vi "img test14(manual vs tracked value).vi"() -> ()   [LabVIEW 2014]
uses:
  <vilib>/Utility/sysdir.llb/System Directory Type.ctl
  <vilib>/Utility/file.llb/Write To Spreadsheet File (string).vi
  <vilib>/vision/NI_Vision_Development_Module.lvlib
panel:
  out "Array of Real World Coordinates 2":cluster{"X":sgl, "Y":sgl}[](array[cluster]) {"Y" format="%.2f"; "X" format="%.2f"}
  out "Array of Real World Coordinates":cluster{"X":sgl, "Y":sgl}[](array[cluster]) {"Y" format="%.2f"; "X" format="%.2f"}
  out "Top VIew 3":cluster{"X":sgl, "Y":sgl}[](graph) caption="Top VIew"
  out "ref points":T1
  out "manual bottom 2":T2[](array[typedef]) {"Y" format="%.2f"; "X" format="%.2f"}
  out "manual top 2":T2[](array[typedef]) {"Y" format="%.2f"; "X" format="%.2f"}
  out "Auto bottom 2":cluster{"Numeric":dbl, "Numeric":dbl}[](array[cluster])
  out "Auto top 2":cluster{"Numeric":dbl, "Numeric":dbl}[](array[cluster])
  out "Auto top":cluster{"Numeric":dbl, "Numeric":dbl}[](array[cluster])
  out "manual bottom":T2[](array[typedef]) {"Y" format="%.2f"; "X" format="%.2f"}
  in  "ON":bool
  in  "STOP":bool
  out "appended array":cluster{"Numeric":dbl, "Numeric":dbl}[](array[cluster])
  out "Top VIew 2":cluster{"X":sgl, "Y":sgl}[](graph) caption="Top VIew"
  out "Auto bottom":cluster{"Numeric":dbl, "Numeric":dbl}[](array[cluster])
  out "Point":T2 {"Y" format="%.2f"; "X" format="%.2f"}
  out "manual top":T2[](array[typedef]) {"Y" format="%.2f"; "X" format="%.2f"}
  out "Number of Frames":u32
  out "Top player court segment display 2":bool[][](array[boolean])
  out "count top":i32[](graph)
  out "count bottom":i32[](graph)
  out "trans top":i32[](graph)
  out "trans bottom":i32[](graph)
  out "trans array bottom":i32[](array[numeric])
  out "trans array top":i32[](array[numeric])
  out "count array bottom":i32[](array[numeric])
  out "Count array top":i32[](array[numeric])
  in  "ON":bool
  out "Top player court segment display":bool[][](array[boolean])
  out "bottom player":cluster{"Numeric":dbl, "Numeric":dbl}[](array[cluster])
  out "top player":cluster{"Numeric":dbl, "Numeric":dbl}[](array[cluster])
  in  "playing":bool
  out "Top VIew":cluster{"Numeric":dbl, "Numeric":dbl}[](graph)
  out "Image 4":T3(plugin-control)
  in  "frame jump":i32=3
  in  "speed":u32(slide)
  in  "start":i32(slide) step=219843704 scale=0.0..62085.0
  out "Image 3":T3(plugin-control)
  in  "AVI Path":path=path "E:/PhD work/PhD research work/Videos/Chen Jin vs Hu Yun (Edited).avi"
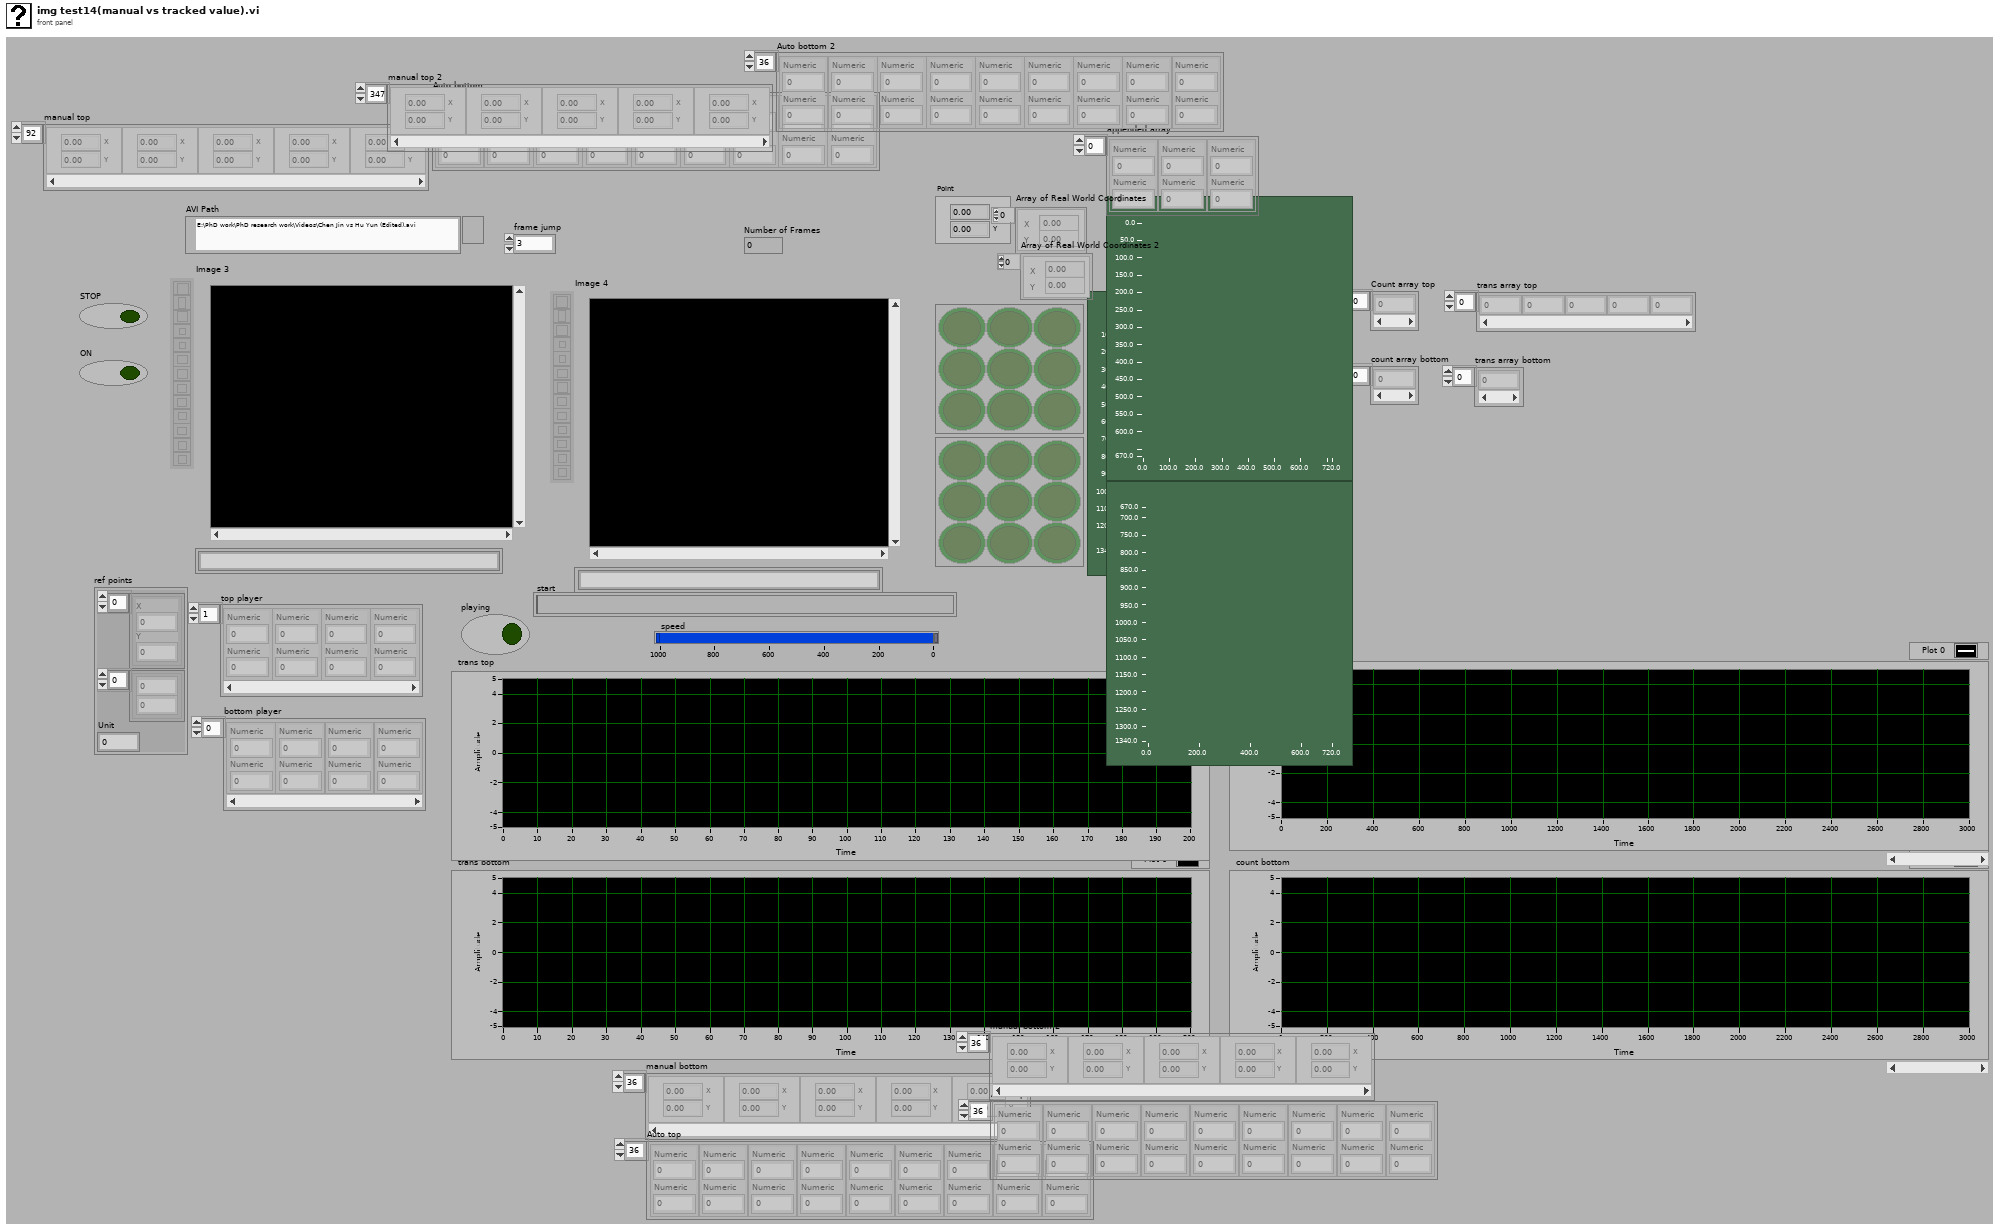
[diagram p1: front panel]
types:
  T1 = cluster{cluster{"X":sgl, "Y":sgl}[], cluster{i32, i32}[], "Unit":u32}
  T2 = typedef "IMAQ Point" = cluster{"X":sgl, "Y":sgl}
  T3 = typedef "IMAQ Image.ctl" = refnum<image>
  T4 = typedef "System Directory Type.ctl" = i32
  T5 = cluster{"Origin Pixel":cluster{"X":sgl, "Y":sgl}, "Angle Relative to Horizontal (deg)":sgl, "Axis Reference":u32}
  T6 = typedef "Image Type" = u32
  T7 = typedef "AviRefnum.ctl" = refnum<k1>
  T8 = cluster{"width":u32, "height":u32, "framesPerSecond":u32, "compressionFilter":string, "hasData":bool}
  T9 = typedef "Particle Parameters" = i32
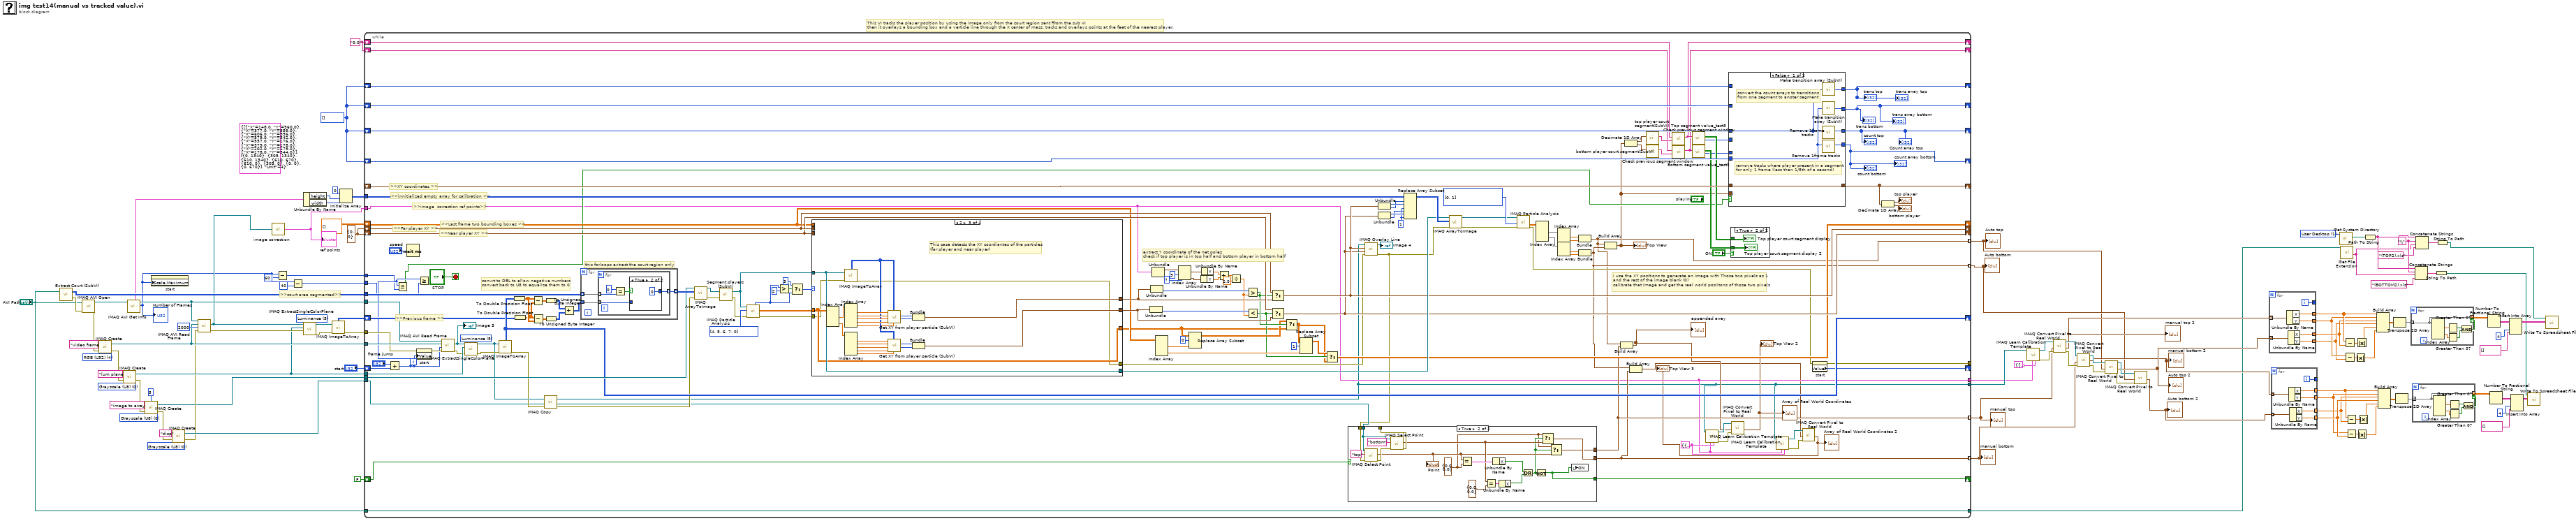
[diagram p0: block diagram]
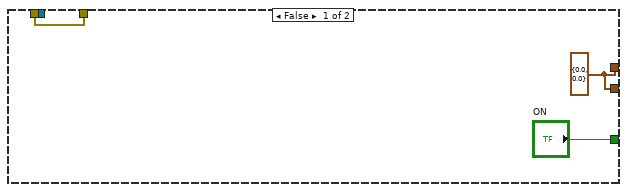
[diagram p2: hidden frame]
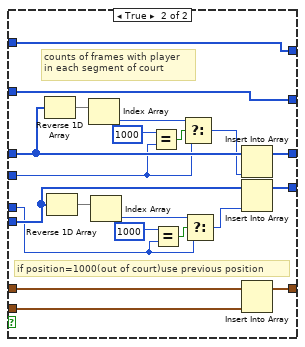
[diagram p3: hidden frame]
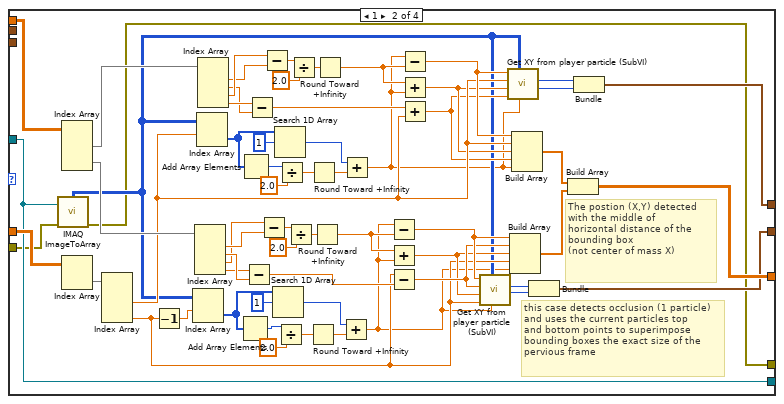
[diagram p6: hidden frame]
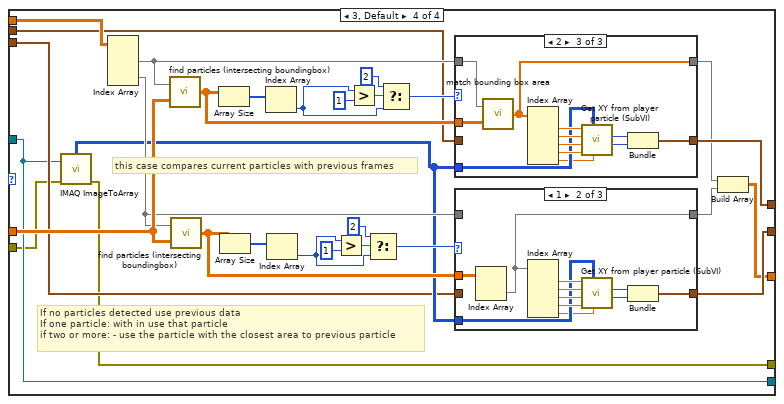
[diagram p7: hidden frame]
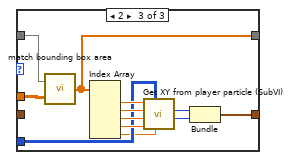
[diagram p9: hidden frame]
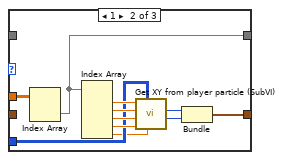
[diagram p11: hidden frame]
diagram:
  w7 = "\\" ("string")
  w17 = T4 1 items=["User Home"=0, "User Desktop"=1, "User Documents"=2, "User Application Data"=3, "User Preferences"=4, "User Temporary"=5, "Public Documents"=6, "Public Application Data"=7, "Public Preferences"=8, "Public Cache"=13, "System Core Libraries"=9, "System Installed Libraries"=10, "Application Files"=11, "Boot Volume Root"=12] ("system directory type")
  (unwired) T1 {[{"X"=148.0, "Y"=560.0}, {"X"=377.0, "Y"=559.0}, {"X"=606.0, "Y"=556.0}, {"X"=579.0, "Y"=342.0}, {"X"=557.0, "Y"=176.0}, {"X"=379.0, "Y"=178.0}, {"X"=202.0, "Y"=179.0}, {"X"=178.0, "Y"=344.0}], [{0, 1340}, {305, 1340}, {610, 1340}, {610, 670}, {610, 0}, {305, 0}, {0, 0}, {0, 670}], "Unit"=4} ("ref points")
  w71 = "0,0" ("Player segment position")
  w72 = i32[] [] ("input array")
  w82 = cluster{"X coordinate":i32, "Y coordinate":i32} {"X coordinate"=0, "Y coordinate"=0}
  w95 = T6 0 items=["Grayscale (U8)", "Grayscale (I16)", "Grayscale (SGL)", "Complex (CSG)", "RGB (U32)", "HSL (U32)", "RGB (U64)", "Grayscale (U16)"] ("Image Type")
  w102 = 5 items=["Red", "Green", "Blue", "Hue", "Saturation", "Luminance", "Value", "Intensity"] ("Color Plane")
  w103 = T6 0 items=["Grayscale (U8)", "Grayscale (I16)", "Grayscale (SGL)", "Complex (CSG)", "RGB (U32)", "HSL (U32)", "RGB (U64)", "Grayscale (U16)"] ("Image Type")
  w107 = T6 0 items=["Grayscale (U8)", "Grayscale (I16)", "Grayscale (SGL)", "Complex (CSG)", "RGB (U32)", "HSL (U32)", "RGB (U64)", "Grayscale (U16)"] ("Image Type")
  w105 = T6 4 items=["Grayscale (U8)", "Grayscale (I16)", "Grayscale (SGL)", "Complex (CSG)", "RGB (U32)", "HSL (U32)", "RGB (U64)", "Grayscale (U16)"] ("Image Type")
  # ">>court area segmented>>"
  # "This VI tracks the player position by using the image only from the court region sent ffrom the sub VI\nthen it overlays a bounding box and a verticle line through the X center of mass. tracks and overlays points at the feet of the nearest player."
  n1 = call "Extract Court (SubVI).vi"("AVI Path"="AVI Path") -> ("error out"=w109:errorcluster, "Court pixels out"=w85:u8[][])  [unwired: 1 in]
  n2 = call "IMAQ AVI Open"("error in (no error)"=w109, "AVI Path"="AVI Path") -> ("error out"=w91:errorcluster, "Avi Refnum"=w80:T7)  [unwired: 8 in]
  n3 = call "IMAQ Create"("Image Name"="video frame", "Image Type"=w105, "error in (no error)"=w91) -> ("New Image"=w99:T3, "error out"=w90:errorcluster)  [unwired: 2 in]
  n4 = call "IMAQ Create"("Image Name"="lum plane", "Image Type"=w107, "error in (no error)"=w90) -> ("New Image"=w98:T3, "error out"=w89:errorcluster)  [unwired: 2 in]
  n5 = call "IMAQ AVI Get Info"("Avi Refnum"=w80) -> ("Number of Frames"=w69:u32, "Avi Refnum (duplicate)"=w79:T7, "Frame Data"=w76:T8)  [unwired: 6 in, 2 out]
  "Number of Frames" <- w69
  n6 = call "IMAQ Create"("Border Size"=5, "Image Name"="image to array", "Image Type"=w103, "error in (no error)"=w89) -> ("New Image"=w84:T3, "error out"=w88:errorcluster)  [unwired: 1 in]
  n7 = property on="start" class="Slide (strict)"("Scale.Maximum"=w69) -> ()  [unwired: 2 in, 2 out]
  n8 = call "IMAQ Create"("Image Name"="disp", "Image Type"=w95, "error in (no error)"=w88) -> ("New Image"=w93:T3, "error out"=w87:errorcluster)  [unwired: 2 in]
  n9 = call "IMAQ AVI Read Frame"("error in (no error)"=w87, "Frame Number"=u32 2000, "Image"=w99, "Avi Refnum"=w79) -> ("error out"=w101:errorcluster, "Image Out"=w70:T3)  [unwired: 4 in, 2 out]
  n10 = call "image correction.vi"("Image"=w70) -> ("ref points"=w1:T1)
  "ref points" <- w1
  n11 = Subtract(x=w69, y=u32 60) -> (x-y=w66:u32)
  n12 = Subtract(x=w69, y=u32 40) -> (x-y=w65:u32)
  n13 = Unbundle By Name(w76) -> ("height"=w75:u32, "width"=w74:u32)
  n14 = call "IMAQ ExtractSingleColorPlane"("Color Plane"=w102, "error in (no error)"=w101, "Image Dst"=w98, "Image Src"=w70) -> ("error out"=w92:errorcluster, "Image Dst Out"=w96:T3)  [unwired: 6 in]
  n15 = call "IMAQ ImageToArray"("error in (no error)"=w92, "Image"=w96) -> ("error out"=w78:errorcluster, "Image Pixels (U8)"=w97:u8[][])  [unwired: 2 in, 3 out]
  n16 = Initialize Array(u8 0 ("element"), w75, w74) -> (w73:u8[][])
  n17 = while {
    tunnel: w79 -> [w219]
    tunnel: w99 -> [w236]
    tunnel: w85 -> [w251]
    tunnel: w98 -> [w237]
    tunnel: w84 -> [w249]
    shift-right: [w248] -> _
    shift-left: w97 -> [w247]
    tunnel: w93 -> [w127]
    shift-right: [w168] -> _
    shift-left: dbl[][] [] ("Particle Measurements (Pixels)") -> [w178]
    shift-right: [w182] -> _
    shift-left: w82 -> [w184]
    shift-right: [w180] -> _
    shift-left: w82 -> [w183]
    shift-right: [w216] -> _
    shift-left: "start" -> [w221]
    tunnel: w78 -> [w218]
    tunnel: w73 -> [w215]
    tunnel: w1 -> [w115]
    shift-right: [w154] -> _
    shift-left: _ -> [w199]
    shift-right: [w152] -> _
    shift-left: w72 -> [w157]
    shift-right: [w151] -> _
    shift-left: w72 -> [w158]
    tunnel: [w160] -> _
    shift-right: [w144] -> _
    shift-left: w72 -> [w155]
    shift-right: [w153] -> _
    shift-left: w72 -> [w156]
    shift-right: [w138] -> _
    shift-left: w71 -> [w145]
    shift-right: [w139] -> _
    shift-left: w71 -> [w146]
    tunnel: w66 -> [w137]
    tunnel: w65 -> [w136]
    tunnel: [w133] -> w5 mode=indexing
    tunnel: [w125] -> w3 mode=indexing
    shift-right: [w129] -> _
    shift-left: FALSE ("ON") -> [w128]
    tunnel: [w123] -> w4 mode=indexing
    tunnel: [w124] -> w2 mode=indexing
    tunnel: [w114] -> w63
    tunnel: [w115] -> w62
    tunnel: "AVI Path" -> [w126]
    tunnel: [w126] -> w15
    stop <- "STOP" stop-if-true
    w116 = T5 {"Origin Pixel"={"X"=-1.0, "Y"=-1.0}, "Angle Relative to Horizontal (deg)"=0.0, "Axis Reference"=1} ("Calibration Axis Info")
    w207 = T9[] [0, 1] items=["Center of Mass X", "Center of Mass Y", "First Pixel X", "First Pixel Y", "Bounding Rect Left", "Bounding Rect Top", "Bounding Rect Right", "Bounding Rect Bottom", "Max Feret Diameter Start X", "Max Feret Diameter Start Y", "Max Feret Diameter End X", "Max Feret Diameter End Y", "Max Horiz. Segment Length Left", "Max Horiz. Segment Length Right", "Max Horiz. Segment Length Row", "-", "Bounding Rect Width", "Bounding Rect Height", "Bounding Rect Diagonal", "Perimeter", "Convex Hull Perimeter", "Holes' Perimeter", "Max Feret Diameter", "Equivalent Ellipse Major Axis", "Equivalent Ellipse Minor Axis", "Equivalent Ellipse Minor Axis (Feret)", "Equivalent Rect Long Side", "Equivalent Rect Short Side", "Equivalent Rect Diagonal", "Equivalent Rect Short Side (Feret)", "Average Horiz. Segment Length", "Average Vert. Segment Length", "Hydraulic Radius", "Waddel Disk Diameter", "-", "Area", "Holes' Area", "Particle & Holes' Area", "Convex Hull Area", "Image Area", "-", "Number of Holes", "Number of Horiz. Segments", "Number of Vert. Segments", "-", "Orientation", "Max Feret Diameter Orientation", "-", "% Area/Image Area", "% Area/(Particle & Holes' Area)", "Ratio of Equivalent Ellipse Axes", "Ratio of Equivalent Rect Sides", "-", "Elongation Factor", "Compactness Factor", "Heywood Circularity Factor", "Type Factor", "-", "Sum X", "Sum Y", "Sum XX", "Sum XY", "Sum YY", "Sum XXX", "Sum XXY", "Sum XYY", "Sum YYY", "-", "Moment of Inertia XX", "Moment of Inertia XY", "Moment of Inertia YY", "Moment of Inertia XXX", "Moment of Inertia XXY", "Moment of Inertia XYY", "Moment of Inertia YYY", "Norm. Moment of Inertia XX", "Norm. Moment of Inertia XY", "Norm. Moment of Inertia YY", "Norm. Moment of Inertia XXX", "Norm. Moment of Inertia XXY", "Norm. Moment of Inertia XYY", "Norm. Moment of Inertia YYY", "Hu Moment 1", "Hu Moment 2", "Hu Moment 3", "Hu Moment 4", "Hu Moment 5", "Hu Moment 6", "Hu Moment 7"] ("Real-World Measurements")
    w210 = u8 1 ("new element/subarray")
    w238 = T9[] [4, 5, 6, 7, 0] items=["Center of Mass X", "Center of Mass Y", "First Pixel X", "First Pixel Y", "Bounding Rect Left", "Bounding Rect Top", "Bounding Rect Right", "Bounding Rect Bottom", "Max Feret Diameter Start X", "Max Feret Diameter Start Y", "Max Feret Diameter End X", "Max Feret Diameter End Y", "Max Horiz. Segment Length Left", "Max Horiz. Segment Length Right", "Max Horiz. Segment Length Row", "-", "Bounding Rect Width", "Bounding Rect Height", "Bounding Rect Diagonal", "Perimeter", "Convex Hull Perimeter", "Holes' Perimeter", "Max Feret Diameter", "Equivalent Ellipse Major Axis", "Equivalent Ellipse Minor Axis", "Equivalent Ellipse Minor Axis (Feret)", "Equivalent Rect Long Side", "Equivalent Rect Short Side", "Equivalent Rect Diagonal", "Equivalent Rect Short Side (Feret)", "Average Horiz. Segment Length", "Average Vert. Segment Length", "Hydraulic Radius", "Waddel Disk Diameter", "-", "Area", "Holes' Area", "Particle & Holes' Area", "Convex Hull Area", "Image Area", "-", "Number of Holes", "Number of Horiz. Segments", "Number of Vert. Segments", "-", "Orientation", "Max Feret Diameter Orientation", "-", "% Area/Image Area", "% Area/(Particle & Holes' Area)", "Ratio of Equivalent Ellipse Axes", "Ratio of Equivalent Rect Sides", "-", "Elongation Factor", "Compactness Factor", "Heywood Circularity Factor", "Type Factor", "-", "Sum X", "Sum Y", "Sum XX", "Sum XY", "Sum YY", "Sum XXX", "Sum XXY", "Sum XYY", "Sum YYY", "-", "Moment of Inertia XX", "Moment of Inertia XY", "Moment of Inertia YY", "Moment of Inertia XXX", "Moment of Inertia XXY", "Moment of Inertia XYY", "Moment of Inertia YYY", "Norm. Moment of Inertia XX", "Norm. Moment of Inertia XY", "Norm. Moment of Inertia YY", "Norm. Moment of Inertia XXX", "Norm. Moment of Inertia XXY", "Norm. Moment of Inertia XYY", "Norm. Moment of Inertia YYY", "Hu Moment 1", "Hu Moment 2", "Hu Moment 3", "Hu Moment 4", "Hu Moment 5", "Hu Moment 6", "Hu Moment 7"] ("Pixel Measurements")
    w252 = 5 items=["Red", "Green", "Blue", "Hue", "Saturation", "Luminance", "Value", "Intensity"] ("Color Plane")
    # ">>XY coordinates >>"
    # ">>innitialized empty array for calibration >>"
    # ">>image  correction ref points>>"
    # "extract Y coordinate of the net poles\ncheck if top player is in top half and bottom player in bottom half"
    # "i use the XY positions to generate an Image with Those two pixels as 1 \nand the rest of the image blank (0)\ncalibrate that image and get the real world posiitons of those two pixels"
    # ">>Last frame two bounding boxes >>"
    # ">>Far player XY >>"
    # ">>Near player XY >>"
    # ">>Previous frame >>"
    # "convrt to DBL to allow negative numbers\nconvert back to U8 to equalize them to 0"
    # "this forloops extract the court region only"
    n18 = Add(x="frame jump", y=w221) -> (x+y=w143:i32)
    n19 = Less Or Equal?(x=w143, y=w137) -> (x <= y?=w142:bool)
    n20 = Wait (ms)(milliseconds to wait="speed") -> ()  [unwired: 1 out]
    n21 = property on="start" class="Slide (strict)"(error in=w218, "Value"=w143) -> (error out=w217:errorcluster)  [unwired: 1 in, 1 out]
    n22 = Greater Or Equal?(x=w143, y=w136) -> ()  [unwired: 1 out]
    n23 = call "IMAQ AVI Read Frame"("error in (no error)"=w217, "Frame Number"=w143, "Image"=w236, "Avi Refnum"=w219) -> ("error out"=w111:errorcluster, "Image Out"=w135:T3)  [unwired: 4 in, 2 out]
    "Image 3" <- w135
    n24 = call "IMAQ ExtractSingleColorPlane"("Color Plane"=w252, "error in (no error)"=w111, "Image Dst"=w237, "Image Src"=w135) -> ("error out"=w239:errorcluster, "Image Dst Out"=w222:T3)  [unwired: 6 in]
    n25 = call "IMAQ ImageToArray"("error in (no error)"=w239, "Image"=w222) -> ("error out"=w164:errorcluster, "Image Pixels (U8)"=w248:u8[][])  [unwired: 2 in, 3 out]
    n26 = To Double Precision Float(number=w248) -> (double precision float=w243:dbl[][])
    n27 = To Double Precision Float(number=w247) -> (double precision float=w242:dbl[][])
    n28 = Subtract(x=w243, y=w242) -> (x-y=w241:dbl[][])
    n29 = Subtract(x=w242, y=w243) -> (x-y=w240:dbl[][])
    n30 = call "IMAQ Copy"("error in (no error)"=w164, "Image Dst"=w127, "Image Src"=w222) -> ("error out"=w163:errorcluster, "Image Dst Out"=w114:T3)  [unwired: 3 in]
    n31 = To Unsigned Byte Integer(number=w241) -> (unsigned 8bit integer=w246:u8[][])
    n32 = To Unsigned Byte Integer(number=w240) -> (unsigned 8bit integer=w245:u8[][])
    n33 = Add(x=w246, y=w245) -> (x+y=w244:u8[][])
    n34 = for {
      tunnel: w251 -> [w474] mode=indexing
      tunnel: [w473] -> w250 mode=indexing
      tunnel: w244 -> [w472] mode=indexing
      n35 = for {
        tunnel: w474 -> [w479] mode=indexing
        tunnel: [w476] -> w473 mode=indexing
        tunnel: w472 -> [w475] mode=indexing
        n36 = Equal?(x=u8 0, y=w479) -> (x = y?=w477:bool)
        n37 = case shown="True" w477 {
          tunnel: [w480 u8 0 ("x")] -> w476
          tunnel: w475 -> [w480 _]
          frame False {
          }
          frame True {
          }
        }
      }
    }
    n38 = call "IMAQ ArrayToImage"("error in (no error)"=w163, "Image Pixels (U8)"=w250, "Image"=w249) -> ("error out"=w234:errorcluster, "Image Out"=w235:T3)  [unwired: 7 in]
    n39 = call "Segment players (SubVI).vi"("error In"=w234, "Image In"=w235) -> ("error out"=w228:errorcluster, "Image Out"=w226:T3)
    n40 = call "IMAQ Particle Analysis"("error in (no error)"=w228, "Pixel Measurements"=w238, "Image"=w226) -> ("error out"=w227:errorcluster, "Particle Measurements (Pixels)"=w225:dbl[][], "Number of Particles"=w230:i32)  [unwired: 3 in, 3 out]
    n41 = Greater?(x=w230, y=2) -> (0:w233:bool)
    n42 = Select(t=3 ("y"), s=w233, f=w230) -> (s? t:f=w229:i32)
    n43 = case shown="2" w229 {
      tunnel: [w307 w334 w388 w398] -> w208
      tunnel: w225 -> [_ w369 w374 w418]
      tunnel: w227 -> [w304 w310 w371 w394]
      tunnel: w226 -> [w307 w334 w388 w398]
      tunnel: [w305 w318 w376 w400] -> w179
      tunnel: [w306 w325 w375 w399] -> w181
      tunnel: [w308 w335 w374 w395] -> w167
      tunnel: w178 -> [w308 w359 _ w421]
      tunnel: w184 -> [w306 _ _ w406]
      tunnel: w183 -> [w305 _ _ w401]
      tunnel: [w304 w309 w370 w393] -> w162
      frame 0 {
        # "This case identifies frames where no particles are detected and keeps the same values from the\nprevious frame"
      }
      frame 1 {
        # "The postion (X,Y) detected with the middle of \nhorizontal distance of the bounding box\n(not center of mass X)"
        # "this case detects occlusion (1 particle)\nand uses the current particles top \nand bottom points to superimpose \nbounding boxes the exact size of the \npervious frame"
        n44 = call "IMAQ ImageToArray"("error in (no error)"=w310, "Image"=w334) -> ("error out"=w309:errorcluster, "Image Pixels (U8)"=w317:u8[][])  [unwired: 2 in, 3 out]
        n45 = Index Array(array=w359) -> (element #1=w367:dbl[], element #2=w339:dbl[])  [unwired: 4 in]
        n46 = Index Array(array=w369) -> (element=w368:dbl[])  [unwired: 2 in]
        n47 = Index Array(array=w368) -> (element #2=w330:dbl, element #4=w321:dbl)  [unwired: 4 in, 2 out]
        n48 = Decrement(x=w321) -> (x-1=w332:dbl)
        n49 = Index Array(array=w317, index (row)=w332) -> (element=w354:u8[])  [unwired: 1 in]
        n50 = Index Array(array=w339) -> (element #1=w343:dbl, element #2=w346:dbl, element #3=w342:dbl, element #4=w345:dbl)  [unwired: 4 in]
        n51 = Index Array(array=w317, index (row)=w330) -> (element=w347:u8[])  [unwired: 1 in]
        n52 = Index Array(array=w367) -> (element #1=w363:dbl, element #2=w360:dbl, element #3=w364:dbl, element #4=w361:dbl)  [unwired: 4 in]
        n53 = Add Array Elements(numeric array=w354) -> (sum=w355:u8)
        n54 = Add Array Elements(numeric array=w347) -> (sum=w351:u8)
        n55 = Subtract(x=w345, y=w346) -> (x-y=w333:dbl)
        n56 = Subtract(x=w361, y=w360) -> (x-y=w338:dbl)
        n57 = Subtract(x=w342, y=w343) -> (x-y=w341:dbl)
        n58 = Subtract(x=w364, y=w363) -> (x-y=w365:dbl)
        n59 = Search 1D Array(1D array=w354, element=u8 1) -> (index of element=w353:i32)  [unwired: 1 in]
        n60 = Search 1D Array(1D array=w347, element=u8 1) -> (index of element=w352:i32)  [unwired: 1 in]
        n61 = Divide(x=w355, y=2.0) -> (x/y=w356:dbl)
        n62 = Divide(x=w351, y=2.0) -> (x/y=w350:dbl)
        n63 = Divide(x=w341, y=2.0) -> (x/y=w344:dbl)
        n64 = Divide(x=w365, y=2.0) -> (x/y=w362:dbl)
        n65 = Round Toward +Infinity(x=w356) -> (ceil(x): smallest int >= x=w315:dbl)
        n66 = Round Toward +Infinity(x=w350) -> (ceil(x): smallest int >= x=w314:dbl)
        n67 = Round Toward +Infinity(x=w344) -> (ceil(x): smallest int >= x=w316:dbl)
        n68 = Round Toward +Infinity(x=w362) -> (ceil(x): smallest int >= x=w313:dbl)
        n69 = Add(x=w353, y=w315) -> (x+y=w311:dbl)
        n70 = Add(x=w352, y=w314) -> (x+y=w312:dbl)
        n71 = Subtract(x=w311, y=w316) -> (x-y=w324:dbl)
        n72 = Add(x=w316, y=w311) -> (x+y=w322:dbl)
        n73 = Subtract(x=w321, y=w333) -> (x-y=w323:dbl)
        n74 = Subtract(x=w312, y=w313) -> (x-y=w331:dbl)
        n75 = Add(x=w313, y=w312) -> (x+y=w329:dbl)
        n76 = Add(x=w338, y=w330) -> (x+y=w328:dbl)
        n77 = call "Get XY from player particle (SubVI).vi"("Center of mass X"=w311, "Image in Pixels (U8)"=w317, "Particle bounding rect bottom"=w321, "Particle bounding rect right"=w322, "Particle bounding rect top"=w323, "Particle bounding rect left"=w324) -> ("Y coordinate"=w319:i32, "X coordinate"=w320:i32)  [unwired: 2 in]
        n78 = call "Get XY from player particle (SubVI).vi"("Center of mass X"=w312, "Image in Pixels (U8)"=w317, "Particle bounding rect bottom"=w328, "Particle bounding rect right"=w329, "Particle bounding rect top"=w330, "Particle bounding rect left"=w331) -> ("Y coordinate"=w326:i32, "X coordinate"=w327:i32)  [unwired: 2 in]
        n79 = Build Array(w324, w323, w322, w321, w311) -> (w336:dbl[])
        n80 = Build Array(w331, w330, w329, w328, w312) -> (w337:dbl[])
        n81 = Bundle("X coordinate"=w320, "Y coordinate"=w319) -> (w318:cluster{"X coordinate":i32, "Y coordinate":i32})  [unwired: 1 in]
        n82 = Build Array(w337, w336) -> (w335:dbl[][])
        n83 = Bundle("X coordinate"=w327, "Y coordinate"=w326) -> (w325:cluster{"X coordinate":i32, "Y coordinate":i32})  [unwired: 1 in]
      }
      frame 2 {
        # "This case detects the XY coordiantes of the particles\n(far player and near player)"
        n84 = Index Array(array=w374) -> (element #1=w382:dbl[], element #2=w381:dbl[])  [unwired: 4 in]
        n85 = call "IMAQ ImageToArray"("error in (no error)"=w371, "Image"=w388) -> ("error out"=w370:errorcluster, "Image Pixels (U8)"=w383:u8[][])  [unwired: 2 in, 3 out]
        n86 = Index Array(array=w382) -> (element #1=w392:dbl, element #2=w391:dbl, element #3=w390:dbl, element #4=w389:dbl, element #5=w373:dbl)  [unwired: 5 in]
        n87 = Index Array(array=w381) -> (element #1=w384:dbl, element #2=w385:dbl, element #3=w386:dbl, element #4=w387:dbl, element #5=w372:dbl)  [unwired: 5 in]
        n88 = call "Get XY from player particle (SubVI).vi"("Center of mass X"=w373, "Image in Pixels (U8)"=w383, "Particle bounding rect bottom"=w389, "Particle bounding rect right"=w390, "Particle bounding rect top"=w391, "Particle bounding rect left"=w392) -> ("Y coordinate"=w379:i32, "X coordinate"=w380:i32)  [unwired: 2 in]
        n89 = call "Get XY from player particle (SubVI).vi"("Center of mass X"=w372, "Image in Pixels (U8)"=w383, "Particle bounding rect bottom"=w387, "Particle bounding rect right"=w386, "Particle bounding rect top"=w385, "Particle bounding rect left"=w384) -> ("Y coordinate"=w377:i32, "X coordinate"=w378:i32)  [unwired: 2 in]
        n90 = Bundle("X coordinate"=w380, "Y coordinate"=w379) -> (w375:cluster{"X coordinate":i32, "Y coordinate":i32})  [unwired: 1 in]
        n91 = Bundle("X coordinate"=w378, "Y coordinate"=w377) -> (w376:cluster{"X coordinate":i32, "Y coordinate":i32})  [unwired: 1 in]
      }
      frame 3, Default {
        # "If no particles detected use previous data\nIf one particle: with in use that particle\nif two or more: - use the particle with the closest area to previous particle"
        # "this case compares current particles with previous frames"
        n92 = call "IMAQ ImageToArray"("error in (no error)"=w394, "Image"=w398) -> ("error out"=w393:errorcluster, "Image Pixels (U8)"=w402:u8[][])  [unwired: 2 in, 3 out]
        n93 = Index Array(array=w421) -> (element #1=w417:dbl[], element #2=w405:dbl[])  [unwired: 4 in]
        n94 = call "find particles (intersecting boundingbox).vi"("Particle Measurements in (bounding boxes)"=w418, "bounding box in"=w417) -> ("Particles within bounding box"=w416:dbl[][])
        n95 = call "find particles (intersecting boundingbox).vi"("Particle Measurements in (bounding boxes)"=w418, "bounding box in"=w405) -> ("Particles within bounding box"=w403:dbl[][])
        n96 = Array Size(array=w416) -> (size(s)=w420:i32[])
        n97 = Array Size(array=w403) -> (size(s)=w419:i32[])
        n98 = Index Array(array=w420) -> (element=w408:i32)  [unwired: 1 in]
        n99 = Index Array(array=w419) -> (element=w409:i32)  [unwired: 1 in]
        n100 = Greater?(x=w409, y=1) -> (0:w412:bool)
        n101 = Greater?(x=w408, y=1) -> (0:w413:bool)
        n102 = Select(t=2 ("y"), s=w412, f=w409) -> (s? t:f=w404:i32)
        n103 = Select(t=2 ("y"), s=w413, f=w408) -> (s? t:f=w407:i32)
        n104 = case shown="2" w407 {
          tunnel: w417 -> [w448 _ w463]
          tunnel: w416 -> [_ w459 w462]
          tunnel: [w448 w450 w461] -> w397
          tunnel: w402 -> [_ w452 w465]
          tunnel: [w447 w451 w464] -> w399
          tunnel: w406 -> [w447 _ _]
          frame 0, Default {
          }
          frame 1 {
            n105 = Index Array(array=w459) -> (element=w450:dbl[])  [unwired: 2 in]
            n106 = Index Array(array=w450) -> (element #1=w456:dbl, element #2=w455:dbl, element #3=w454:dbl, element #4=w453:dbl, element #5=w449:dbl)  [unwired: 5 in]
            n107 = call "Get XY from player particle (SubVI).vi"("Center of mass X"=w449, "Image in Pixels (U8)"=w452, "Particle bounding rect bottom"=w453, "Particle bounding rect right"=w454, "Particle bounding rect top"=w455, "Particle bounding rect left"=w456) -> ("Y coordinate"=w457:i32, "X coordinate"=w458:i32)  [unwired: 2 in]
            n108 = Bundle("X coordinate"=w458, "Y coordinate"=w457) -> (w451:cluster{"X coordinate":i32, "Y coordinate":i32})  [unwired: 1 in]
          }
          frame 2 {
            n109 = call "match bounding box area.vi"("particle measurements (bounding box)"=w462, "bounding box in"=w463) -> ("matching bounding box"=w461:dbl[])
            n110 = Index Array(array=w461) -> (element #1=w469:dbl, element #2=w468:dbl, element #3=w467:dbl, element #4=w466:dbl, element #5=w460:dbl)  [unwired: 5 in]
            n111 = call "Get XY from player particle (SubVI).vi"("Center of mass X"=w460, "Image in Pixels (U8)"=w465, "Particle bounding rect bottom"=w466, "Particle bounding rect right"=w467, "Particle bounding rect top"=w468, "Particle bounding rect left"=w469) -> ("Y coordinate"=w470:i32, "X coordinate"=w471:i32)  [unwired: 2 in]
            n112 = Bundle("X coordinate"=w471, "Y coordinate"=w470) -> (w464:cluster{"X coordinate":i32, "Y coordinate":i32})  [unwired: 1 in]
          }
        }
        n113 = case shown="1" w404 {
          tunnel: w405 -> [w423 _ w438]
          tunnel: w403 -> [_ w434 w437]
          tunnel: [w423 w425 w436] -> w396
          tunnel: w402 -> [_ w427 w440]
          tunnel: [w422 w426 w439] -> w400
          tunnel: w401 -> [w422 _ _]
          frame 0, Default {
          }
          frame 1 {
            n114 = Index Array(array=w434) -> (element=w425:dbl[])  [unwired: 2 in]
            n115 = Index Array(array=w425) -> (element #1=w431:dbl, element #2=w430:dbl, element #3=w429:dbl, element #4=w428:dbl, element #5=w424:dbl)  [unwired: 5 in]
            n116 = call "Get XY from player particle (SubVI).vi"("Center of mass X"=w424, "Image in Pixels (U8)"=w427, "Particle bounding rect bottom"=w428, "Particle bounding rect right"=w429, "Particle bounding rect top"=w430, "Particle bounding rect left"=w431) -> ("Y coordinate"=w432:i32, "X coordinate"=w433:i32)  [unwired: 2 in]
            n117 = Bundle("X coordinate"=w433, "Y coordinate"=w432) -> (w426:cluster{"X coordinate":i32, "Y coordinate":i32})  [unwired: 1 in]
          }
          frame 2 {
            n118 = call "match bounding box area.vi"("particle measurements (bounding box)"=w437, "bounding box in"=w438) -> ("matching bounding box"=w436:dbl[])
            n119 = Index Array(array=w436) -> (element #1=w444:dbl, element #2=w443:dbl, element #3=w442:dbl, element #4=w441:dbl, element #5=w435:dbl)  [unwired: 5 in]
            n120 = call "Get XY from player particle (SubVI).vi"("Center of mass X"=w435, "Image in Pixels (U8)"=w440, "Particle bounding rect bottom"=w441, "Particle bounding rect right"=w442, "Particle bounding rect top"=w443, "Particle bounding rect left"=w444) -> ("Y coordinate"=w445:i32, "X coordinate"=w446:i32)  [unwired: 2 in]
            n121 = Bundle("X coordinate"=w446, "Y coordinate"=w445) -> (w439:cluster{"X coordinate":i32, "Y coordinate":i32})  [unwired: 1 in]
          }
        }
        n122 = Build Array(w397, w396) -> (w395:dbl[][])
      }
    }
    n123 = Unbundle(w179) -> ("Y coordinate"=w186:i32)  [unwired: 1 out]
    n124 = Unbundle(w181) -> ("Y coordinate"=w187:i32)  [unwired: 1 out]
    n125 = Unbundle(w115) -> (w196:cluster{"X":sgl, "Y":sgl}[])  [unwired: 2 out]
    n126 = Index Array(array=w178) -> (element #1=w176:dbl[], element #2=w172:dbl[])  [unwired: 4 in]
    n127 = Index Array(array=w196, index #1=3 ("index"), index #2=7 ("index")) -> (element #1=w193:cluster{"X":sgl, "Y":sgl}, element #2=w192:cluster{"X":sgl, "Y":sgl})
    n128 = Replace Array Subset(array=w167, new element=w176, index (row)=0) -> (w175:dbl[][])  [unwired: 1 in]
    n129 = Unbundle By Name(w192) -> ("Y"=w190:sgl)
    n130 = Unbundle By Name(w193) -> ("Y"=w191:sgl)
    n131 = Add(x=w191, y=w190) -> (x+y=w189:sgl)
    n132 = Divide(x=w189, y=sgl 2.0) -> (x/y=w185:sgl)
    n133 = Greater?(x=w187, y=w185) -> (0:w177:bool)
    n134 = Less?(x=w186, y=w185) -> (x < y?=w170:bool)
    n135 = Select(t=w184, s=w177, f=w181) -> (s? t:f=w182:cluster{"X coordinate":i32, "Y coordinate":i32})
    n136 = Select(t=w183, s=w170, f=w179) -> (s? t:f=w180:cluster{"X coordinate":i32, "Y coordinate":i32})
    n137 = Select(t=w175, s=w177, f=w167) -> (s? t:f=w169:dbl[][])
    n138 = Replace Array Subset(array=w169, new element=w172, index (row)=1) -> (w171:dbl[][])  [unwired: 1 in]
    n139 = Select(t=w171, s=w170, f=w169) -> (s? t:f=w168:dbl[][])
    n140 = call "IMAQ Overlay Line"("error in (no error)"=w162, "End Point"=w180, "Start Point"=w182, "Image"=w114) -> ("error out"=w110:errorcluster, "Image Out"=→"Image 4":T3)  [unwired: 6 in]
    n141 = case shown="True" w128 {
      tunnel: w127 -> [_ w269]
      tunnel: w110 -> [w255 w273]
      tunnel: [w255 w270] -> _
      tunnel: [w253 w258] -> w133
      tunnel: ["ON" w260] -> w129
      tunnel: [w253 w261] -> w123
      frame False {
        w253 = T2 {"X"=0.0, "Y"=0.0} ("Point 2")
      }
      frame True {
        w256 = T2 {"X"=0.0, "Y"=0.0} ("Point 2")
        n142 = call "IMAQ Select Point"("error in (no error)"=w273, "Prompt"="top", "Image In"=w269) -> ("error out"=w271:errorcluster, "Point"=w259:T2)  [unwired: 5 in, 2 out]
        "Point" <- w259
        n143 = call "IMAQ Select Point"("error in (no error)"=w271, "Prompt"="bottom", "Image In"=w269) -> ("error out"=w270:errorcluster, "Point"=w262:T2)  [unwired: 5 in, 2 out]
        n144 = Equal?(x=w259, y=w256) -> (x = y?=w272:cluster{"X":bool, "Y":bool})
        n145 = Equal?(x=w262, y=T2 {"X"=0.0, "Y"=0.0} ("Point 2")) -> (x = y?=w265:cluster{"X":bool, "Y":bool})
        n146 = Unbundle By Name(w272) -> ("X"=w264:bool)
        n147 = Unbundle By Name(w265) -> ("X"=w263:bool)
        n148 = Or(x=w264, y=w263) -> (x .or. y?=w257:bool)
        n149 = Not(x=w257) -> (.not. x?=w260:bool)
        n150 = Select(t=w256, s=w257, f=w262) -> (s? t:f=w261:T2)
        n151 = Select(t=w256, s=w257, f=w259) -> (s? t:f=w258:T2)
        n152 = local write "ON"(w260) -> ()
      }
    }
    n153 = Unbundle(w180) -> ("X coordinate"=w211:i32, "Y coordinate"=w212:i32)
    n154 = Unbundle(w182) -> ("X coordinate"=w214:i32, "Y coordinate"=w213:i32)
    n155 = Replace Array Subset(array=w215, new element #1=w210, index (row) #1=w213, index (col) #1=w214, new element #2=w210, index (row) #2=w212, index (col) #2=w211) -> (w209:u8[][])
    n156 = call "IMAQ ArrayToImage"("error in (no error)"=w110, "Image Pixels (U8)"=w209, "Image"=w208) -> ("error out"=w131:errorcluster, "Image Out"=w132:T3)  [unwired: 7 in]
    n157 = call "IMAQ Particle Analysis"("error in (no error)"=w131, "Real-World Measurements"=w207, "Image"=w132) -> ("error out"=w161:errorcluster, "Particle Measurements (Real-World)"=w206:dbl[][])  [unwired: 3 in, 4 out]
    n158 = Index Array(array=w206) -> (element #1=w205:dbl[], element #2=w204:dbl[])  [unwired: 4 in]
    n159 = Index Array(array=w205) -> (element #1=w201:dbl, element #2=w200:dbl)  [unwired: 2 in]
    n160 = Index Array(array=w204) -> (element #1=w202:dbl, element #2=w203:dbl)  [unwired: 2 in]
    n161 = Bundle("Numeric"=w201, "Numeric"=w200) -> (w124:cluster{"Numeric":dbl, "Numeric":dbl})  [unwired: 1 in]
    n162 = Bundle("Numeric"=w202, "Numeric"=w203) -> (w125:cluster{"Numeric":dbl, "Numeric":dbl})  [unwired: 1 in]
    n163 = Build Array(w124, w125) -> (w134:cluster{"Numeric":dbl, "Numeric":dbl}[])
    "Top VIew" <- w134
    n164 = Build Array(w124, w133) -> (w120:cluster{"Numeric":dbl, "Numeric":dbl}[])
    "appended array" <- w120
    n165 = Decimate 1D Array(w134) -> (w165:cluster{"Numeric":dbl, "Numeric":dbl}[], w166:cluster{"Numeric":dbl, "Numeric":dbl}[])
    n166 = Build Array(w125, w123) -> (w113:cluster{"Numeric":dbl, "Numeric":dbl}[])
    n167 = call "top player court segment(SubVI).vi"("Top player position"=w165) -> ("Top player segment position"=w141:string)  [unwired: 10 in]
    n168 = call "bottom player court segment(SubVI).vi"("Bottom player position"=w166) -> ("Bottom player segment position"=w140:string)  [unwired: 10 in]
    n169 = call "Check previous segment window.vi"("Current player segment position"=w141, "Previous player segment position"=w146) -> ("Player segment position"=w139:string)  [unwired: 9 in]
    n170 = call "Check previous segment window.vi"("Current player segment position"=w140, "Previous player segment position"=w145) -> ("Player segment position"=w138:string)  [unwired: 9 in]
    n171 = call "Top segment value_test3.vi"("Top player segment position"=w139) -> ("Top player segment value"=w149:i32, "Top player court segment display"=w150:bool[][])  [unwired: 9 in]
    n172 = call "Bottom segment value_test3.vi"("Bottom player segment position"=w138) -> ("Bottom player segment"=w147:i32, "Bottom player court segment display"=w148:bool[][])  [unwired: 9 in]
    n173 = call "IMAQ Learn Calibration Template"("Calibration Axis Info"=w116, "Reference Points"=w115, "Image"=w114) -> ("error out"=w122:errorcluster, "Calibrated Image"=w121:T3)  [unwired: 6 in, 1 out]
    n174 = case shown="False" w142 {
      tunnel: w199 -> [w280 w301]
      tunnel: w134 -> [_ w300]
      tunnel: w158 -> [w277 w294]
      tunnel: w157 -> [w276 w284]
      tunnel: [w278 w295] -> w144
      tunnel: [w279 w296] -> w153
      tunnel: w147 -> [_ w281]
      tunnel: w149 -> [_ w289]
      tunnel: w156 -> [_ w296]
      tunnel: w155 -> [_ w295]
      tunnel: [w275 w299] -> w152
      tunnel: [w274 w298] -> w151
      tunnel: [w280 w297] -> w154
      frame False {
        # "convert the count arrays to transitions \nfrom one segment to anoter segment"
        # "remove tracks where player present in a segment \nfor only 1 frame (less than 1/5th of a second)"
        n175 = call "Make transition array (SubVI).vi"("count array in"=w277) -> ("Transition array out"=w278:i32[])
        n176 = call "Make transition array (SubVI).vi"("count array in"=w276) -> ("Transition array out"=w279:i32[])
        n177 = call "Remove 1frame tracks.vi"("count array in"=w277) -> ("count array out"=w274:i32[])  [unwired: 10 in]
        n178 = call "Remove 1frame tracks.vi"("count array in"=w276) -> ("count array out"=w275:i32[])  [unwired: 10 in]
      }
      frame True {
        # "if position=1000(out of court)use previous position"
        # "counts of frames with player\nin each segment of court"
        n179 = Reverse 1D Array(array=w294) -> (reversed array=w293:i32[])
        n180 = Reverse 1D Array(array=w284) -> (reversed array=w283:i32[])
        n181 = Index Array(array=w293) -> (element=w290:i32)  [unwired: 1 in]
        n182 = Index Array(array=w283) -> (element=w287:i32)  [unwired: 1 in]
        n183 = Equal?(x=1000 ("y"), y=w289) -> (x = y?=w291:bool)
        n184 = Equal?(x=1000 ("y"), y=w281) -> (x = y?=w286:bool)
        n185 = Select(t=w290, s=w291, f=w289) -> (s? t:f=w288:i32)
        n186 = Select(t=w287, s=w286, f=w281) -> (s? t:f=w282:i32)
        n187 = Insert Into Array(array=w294, new element=w288) -> (w298:i32[])  [unwired: 1 in]
        n188 = Insert Into Array(array=w284, new element=w282) -> (w299:i32[])  [unwired: 1 in]
        n189 = Insert Into Array(array=w301, new element=w300) -> (w297:cluster{"Numeric":dbl, "Numeric":dbl}[])  [unwired: 1 in]
      }
    }
    "Count array top" <- w151
    "count array bottom" <- w152
    "trans array top" <- w144
    "trans array bottom" <- w153
    "trans bottom" <- w153
    "trans top" <- w144
    "count bottom" <- w152
    "count top" <- w151
    n190 = case shown="True" "ON" {
      tunnel: w150 -> [_ w303]
      tunnel: w148 -> [_ w302]
      frame False {
      }
      frame True {
        "Top player court segment display" <- w303
        "Top player court segment display 2" <- w302
      }
    }
    n191 = call "IMAQ Convert Pixel to Real World"("error in (no error)"=w122, "Array of Pixel Coordinates"=w120, "Calibrated Image"=w121) -> ("Array of Real World Coordinates"=→"Top VIew 2" →"Array of Real World Coordinates":cluster{"X":sgl, "Y":sgl}[])  [unwired: 3 in, 5 out]
    n192 = call "IMAQ Learn Calibration Template"("Calibration Axis Info"=w116, "Reference Points"=w115, "Image"=w114) -> ("error out"=w117:errorcluster, "Calibrated Image"=w118:T3)  [unwired: 6 in, 1 out]
    n193 = call "IMAQ Convert Pixel to Real World"("error in (no error)"=w117, "Array of Pixel Coordinates"=w113, "Calibrated Image"=w118) -> ("Array of Real World Coordinates"=→"Top VIew 3" →"Array of Real World Coordinates 2":cluster{"X":sgl, "Y":sgl}[])  [unwired: 3 in, 5 out]
    n194 = property on="start" class="Slide (strict)"(error in=w161) -> (error out=w160:errorcluster, "Value"=w216:i32)  [unwired: 1 in, 1 out]
    n195 = Decimate 1D Array(w154) -> (→"top player":cluster{"Numeric":dbl, "Numeric":dbl}[], →"bottom player":cluster{"Numeric":dbl, "Numeric":dbl}[])
  }
  "manual top" <- w5
  "Auto bottom" <- w3
  "manual bottom" <- w4
  "Auto top" <- w2
  n196 = call "IMAQ Learn Calibration Template"("Calibration Axis Info"=T5 {"Origin Pixel"={"X"=-1.0, "Y"=-1.0}, "Angle Relative to Horizontal (deg)"=0.0, "Axis Reference"=1}, "Reference Points"=w62, "Image"=w63) -> ("error out"=w56:errorcluster, "Calibrated Image"=w60:T3)  [unwired: 6 in, 1 out]
  n197 = call "IMAQ Convert Pixel to Real World"("error in (no error)"=w56, "Array of Pixel Coordinates"=w5, "Calibrated Image"=w60) -> ("error out"=w55:errorcluster, "Array of Real World Coordinates"=w37:cluster{"X":sgl, "Y":sgl}[], "Calibrated Image (duplicate)"=w59:T3)  [unwired: 3 in, 3 out]
  "manual top 2" <- w37
  n198 = call "IMAQ Convert Pixel to Real World"("error in (no error)"=w55, "Array of Pixel Coordinates"=w4, "Calibrated Image"=w59) -> ("error out"=w54:errorcluster, "Array of Real World Coordinates"=w20:cluster{"X":sgl, "Y":sgl}[], "Calibrated Image (duplicate)"=w58:T3)  [unwired: 3 in, 3 out]
  "manual bottom 2" <- w20
  n199 = call "IMAQ Convert Pixel to Real World"("error in (no error)"=w54, "Array of Pixel Coordinates"=w2, "Calibrated Image"=w58) -> ("error out"=w53:errorcluster, "Array of Real World Coordinates"=w36:cluster{"X":sgl, "Y":sgl}[], "Calibrated Image (duplicate)"=w57:T3)  [unwired: 3 in, 3 out]
  "Auto top 2" <- w36
  n200 = call "IMAQ Convert Pixel to Real World"("error in (no error)"=w53, "Array of Pixel Coordinates"=w3, "Calibrated Image"=w57) -> ("Array of Real World Coordinates"=w19:cluster{"X":sgl, "Y":sgl}[])  [unwired: 3 in, 5 out]
  "Auto bottom 2" <- w19
  n201 = for {
    tunnel: w36 -> [w488] mode=indexing
    tunnel: [w486] -> w49 mode=indexing
    tunnel: [w484] -> w47 mode=indexing
    tunnel: w37 -> [w487] mode=indexing
    tunnel: [w485] -> w50 mode=indexing
    tunnel: [w483] -> w48 mode=indexing
    tunnel: [w482] -> _
    i -> [w482]
    n202 = Unbundle By Name(w487) -> ("X"=w485:sgl, "Y"=w483:sgl)
    n203 = Unbundle By Name(w488) -> ("X"=w486:sgl, "Y"=w484:sgl)
  }
  n204 = for {
    tunnel: w19 -> [w495] mode=indexing
    tunnel: [w493] -> w24 mode=indexing
    tunnel: [w491] -> w26 mode=indexing
    tunnel: w20 -> [w494] mode=indexing
    tunnel: [w492] -> w23 mode=indexing
    tunnel: [w490] -> w25 mode=indexing
    tunnel: [w489] -> _
    i -> [w489]
    n205 = Unbundle By Name(w494) -> ("X"=w492:sgl, "Y"=w490:sgl)
    n206 = Unbundle By Name(w495) -> ("X"=w493:sgl, "Y"=w491:sgl)
  }
  n207 = call <vilib>:"Get System Directory.vi"("system directory type"=w17) -> ("system directory"=w16:path)  [unwired: 10 in]
  n208 = call <vilib>:"Get File Extension.vi"("file"=w15) -> ("filename without extension"=w6:string)  [unwired: 7 in, 3 out]
  n209 = Subtract(x=w50, y=w49) -> (x-y=w46:sgl[])
  n210 = Subtract(x=w48, y=w47) -> (x-y=w45:sgl[])
  n211 = Subtract(x=w23, y=w24) -> (x-y=w27:sgl[])
  n212 = Subtract(x=w25, y=w26) -> (x-y=w28:sgl[])
  n213 = Absolute Value(x=w45) -> (abs(x)=w43:sgl[])
  n214 = Absolute Value(x=w46) -> (abs(x)=w44:sgl[])
  n215 = Absolute Value(x=w28) -> (abs(x)=w30:sgl[])
  n216 = Absolute Value(x=w27) -> (abs(x)=w29:sgl[])
  n217 = Path To String(path=w16) -> (string=w10:string)
  n218 = Build Array(w50, w48, w49, w47, w44, w43) -> (w52:sgl[][])
  n219 = Build Array(w23, w25, w24, w26, w29, w30) -> (w21:sgl[][])
  n220 = Transpose 2D Array(2D array=w52) -> (transposed array=w51:sgl[][])
  n221 = Transpose 2D Array(2D array=w21) -> (transposed array=w22:sgl[][])
  n222 = for {
    tunnel: w51 -> [w498] mode=indexing
    tunnel: [w498] -> w42 mode=indexing if=w499
    n223 = Index Array(array=w498) -> (element #1=w497:sgl, element #3=w496:sgl)  [unwired: 4 in, 2 out]
    n224 = Greater Than 0?(x=w497) -> (x > 0?=w501:bool)
    n225 = Greater Than 0?(x=w496) -> (x > 0?=w500:bool)
    n226 = And(x=w501, y=w500) -> (x .and. y?=w499:bool)
  }
  n227 = for {
    tunnel: w22 -> [w504] mode=indexing
    tunnel: [w504] -> w31 mode=indexing if=w505
    n228 = Index Array(array=w504) -> (element #1=w503:sgl, element #3=w502:sgl)  [unwired: 4 in, 2 out]
    n229 = Greater Than 0?(x=w503) -> (x > 0?=w507:bool)
    n230 = Greater Than 0?(x=w502) -> (x > 0?=w506:bool)
    n231 = And(x=w507, y=w506) -> (x .and. y?=w505:bool)
  }
  n232 = Concatenate Strings(w10, w7, w6, "(BOTTOM2).xls" ("replace string (\"\")")) -> (w11:string)
  n233 = Concatenate Strings(w10, w7, w6, "(TOP2).xls" ("replace string (\"\")")) -> (w14:string)
  n234 = String To Path(string=w11) -> (path=w9:path)
  n235 = String To Path(string=w14) -> (path=w8:path)
  n236 = Number To Fractional String(number=w42) -> (F-format string=w41:string[][])  [unwired: 3 in]
  n237 = Number To Fractional String(number=w31) -> (F-format string=w32:string[][])  [unwired: 3 in]
  n238 = Insert Into Array(array=w41, index (col)=4 ("disabled index (col)"), new element=string[] [] ("new element/subarray")) -> (w38:string[][])  [unwired: 1 in]
  n239 = Insert Into Array(array=w32, index (col)=4 ("disabled index (col)"), new element=string[] [] ("new element/subarray")) -> (w35:string[][])  [unwired: 1 in]
  n240 = call-poly <vilib>:"Write To Spreadsheet File.vi"("2D data"=w35, "file path (dialog if empty)"=w9) -> ()  [unwired: 6 in, 1 out]
  n241 = call-poly <vilib>:"Write To Spreadsheet File.vi"("2D data"=w38, "file path (dialog if empty)"=w8) -> ()  [unwired: 6 in, 1 out]
